vi "SetRGBA.vi"(0 "ColorRGBA in":refnum<class "ColorRGBA.lvclass">, 5 "R":u8, 7 "G":u8, 9 "B":u8, 11 "error in (no error)":errorcluster, 12 "A":u8) -> (4 "ColorRGBA out":refnum<class "ColorRGBA.lvclass">, 15 "error out":errorcluster)   [LabVIEW 2021, in "Picture2D.lvlib" / "ColorRGBA.lvclass"]
uses:
  ColorRGBA.lvclass
  ColorRGBA.lvclass/ColorRGBA.ctl
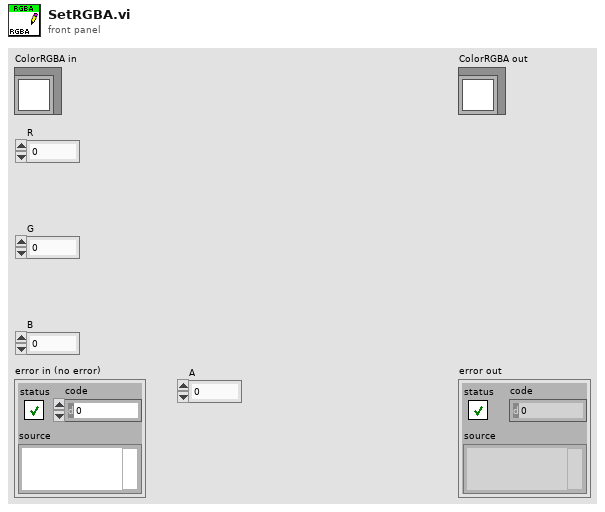
[diagram p1: front panel]
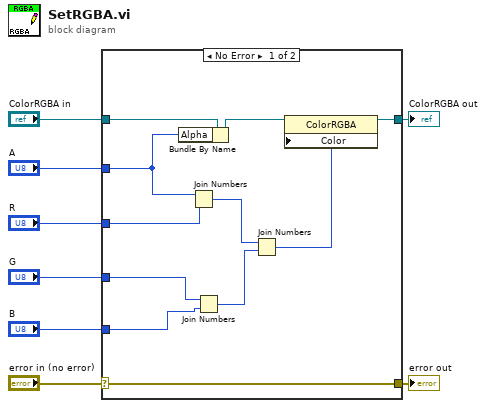
[diagram p0: block diagram]
diagram:
  n1 = case shown="No Error" "error in (no error)" {
    selector: "error in (no error)" -> [w18 w21]
    tunnel: [w18 w21] -> w7
    tunnel: [w16 w20] -> w5
    tunnel: "ColorRGBA in" -> [w19 w20]
    tunnel: "A" -> [w13 _]
    tunnel: "R" -> [w12 _]
    tunnel: "G" -> [w14 _]
    tunnel: "B" -> [w15 _]
    frame No Error {
      n2 = Bundle By Name(cluster=w19, "Alpha"=w13) -> (w17:refnum<class "ColorRGBA.lvclass">)
      n3 = Join Numbers(hi=w13, lo=w12) -> ((hi.lo)=w10:u16)
      n4 = Join Numbers(hi=w14, lo=w15) -> ((hi.lo)=w11:u16)
      n5 = Join Numbers(hi=w10, lo=w11) -> ((hi.lo)=w9:u32)
      n6 = property class="ColorRGBA"(reference=w17, "Color"=w9) -> (reference out=w16:refnum<class "ColorRGBA.lvclass">)  [unwired: 1 in, 1 out]
    }
    frame Error {
    }
  }
  "error out" <- w7
  "ColorRGBA out" <- w5
